vi "Main.vi"(11 "Module Admin":refnum<class "Delacor_lib_QMH_Module Admin.lvclass">) -> ()   [LabVIEW 2026, in "Launcher.lvlib"]
doc: "This template is based off of the Queued Message Handler design pattern and the Queued Message Handler project template that ships with LabVIEW.\n\nThe main difference is that the queue is private to this module and communication between modules is performed via Broadcast and Request events.\n\nRequest events are wrapped in public API methods and are handled in the Event Handling Loop (EHL) of this VI. Any module can register for Broadcast events sent by this module. The EHL generates messages based on user interface actions.\n\nThe Message Handling Loop (MHL) processes messages generated by the EHL, or by other messages. The messages are string values, so new messages can be added easily to the Message Cases case structure in the MHL. Each message cluster can also provide an optional value for Message Data, which is a variant that can be converted to whatever message-specific data is required.\n_____\nBased on DQMH Dev Tools: Project Template 7.1.2.1547."
uses:
  Launcher.lvlib
  <vilib>/Delacor/Delacor QMH/Libraries/Module Admin_class/Delacor_lib_QMH_Module Admin.lvclass
  Module Data--cluster.ctl
  Capture detection loop data--cluster.ctl
  <vilib>/Delacor/Delacor QMH/Libraries/Message Queue_class/Delacor_lib_QMH_Message Queue.lvclass/Delacor_lib_QMH_Message Queue.ctl
  Stop Argument--cluster.ctl
  <vilib>/Delacor/Delacor QMH/Libraries/Module Admin_class/Delacor_lib_QMH_Module Admin.lvclass/Delacor_lib_QMH_Module Admin.ctl
  Set Captures Folder Argument--cluster.ctl
  Set Capture Detection Loop Timeout Argument--cluster.ctl
  Trigger Capture Detection Loop Argument--cluster.ctl
  Trigger Capture Detection Loop (Reply Payload)--cluster.ctl
  <vilib>/Utility/miscctls.llb/LVPointTypeDef.ctl
  <vilib>/Delacor/Delacor QMH/Libraries/Message Queue_class/Delacor_lib_QMH_Enqueue Message (Single).vi
  <vilib>/Delacor/Delacor QMH/Libraries/Module Admin_class/Delacor_lib_QMH_Get External Launch.vi
  <vilib>/Delacor/Delacor QMH/Libraries/Message Queue_class/Delacor_lib_QMH_Message Queue.lvclass
  Core/Core.lvlib
panel:
  out "error out":errorcluster
  out "Status":string
  in  "Simulate MHL Error":bool
  in  "Simulate EHL Error":bool
  # "Other processes communicate with this Module via its Public API (wrappers for its Request Events).\n\nThis Module communicates with other processes via its Broadcast Events.\nAny process that wants to receive these messages can register for this module's Broadcast events."
  # "This template is for the DQMH framework. See the block diagram for more information on how to use this template."
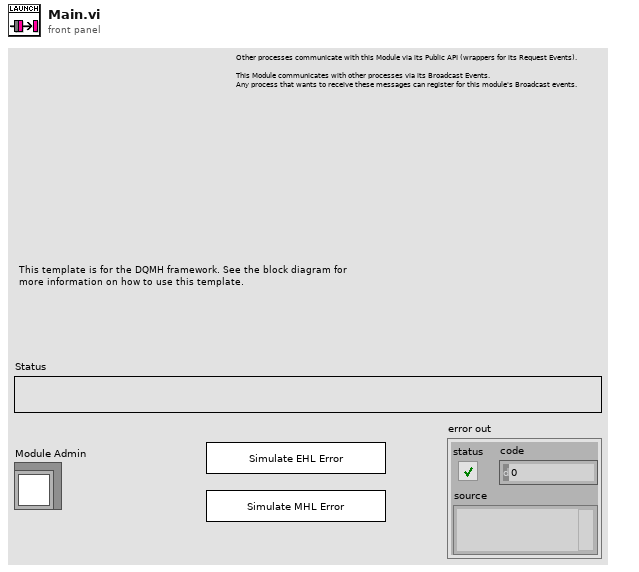
[diagram p1: front panel]
types:
  T1 = typedef "Launcher.lvlib/Broadcast Events--cluster.ctl" = cluster{"Module Did Init":refnum<user-event>, "Status Updated":refnum<user-event>, "Error Reported":refnum<user-event>, "Module Did Stop":refnum<user-event>, "Update Module Execution Status":refnum<user-event>, "Start Capture Detection Loop":refnum<user-event>, "Benchmark Started":refnum<user-event>, "Broadcast number of frames and run ID":refnum<user-event>}
  T2 = typedef "Launcher.lvlib/Request Events--cluster.ctl" = cluster{"Stop Module":refnum<user-event>, "Show Panel":refnum<user-event>, "Hide Panel":refnum<user-event>, "Get Module Execution Status":refnum<user-event>, "Show Diagram":refnum<user-event>, "Set Captures Folder":refnum<user-event>, "Set Capture Detection Loop Timeout":refnum<user-event>, "Trigger Capture Detection Loop":refnum<user-event>}
  T3 = typedef "Capture detection loop data--cluster.ctl" = cluster{"Captures":path, "Timeout":i32, "Reset":bool, "Trigger":bool, "Iteration":i32, "Capture":path}
  T4 = typedef "Launcher.lvlib/Module Data--cluster.ctl" = cluster{"Status":string, "Captures":path, "Capture Detection Loop Timeout":i32}
  T5 = enum32{"invalid lock state", "Not Locked", "Locked (No Password)", "Password-protected"}
  T6 = typedef "Launcher.lvlib/Stop Argument--cluster.ctl" = cluster{"Origin":string, "Exit via Stop Module Req?":bool, "Wait for Module to stop?":bool}
  T7 = typedef "Launcher.lvlib/Set Captures Folder Argument--cluster.ctl" = cluster{"Captures":path}
  T8 = typedef "Launcher.lvlib/Set Capture Detection Loop Timeout Argument--cluster.ctl" = cluster{"Timeout":i32}
  T9 = typedef "Launcher.lvlib/Trigger Capture Detection Loop Argument--cluster.ctl" = cluster{"Capture Detection Loop Timeout":i32, "Wait Notifier":refnum<notifier>, "wait for reply":bool}
  T10 = typedef "LVPointTypeDef.ctl" = cluster{"Horizontal":i16, "Vertical":i16}
  T11 = enum32{"Invalid", "Standard", "Closed", "Hidden", "Minimized", "Maximized"}
  T12 = typedef "Launcher.lvlib/Trigger Capture Detection Loop (Reply Payload)--cluster.ctl" = cluster{"Module Initial Time Stamp":timestamp, "error":errorcluster}
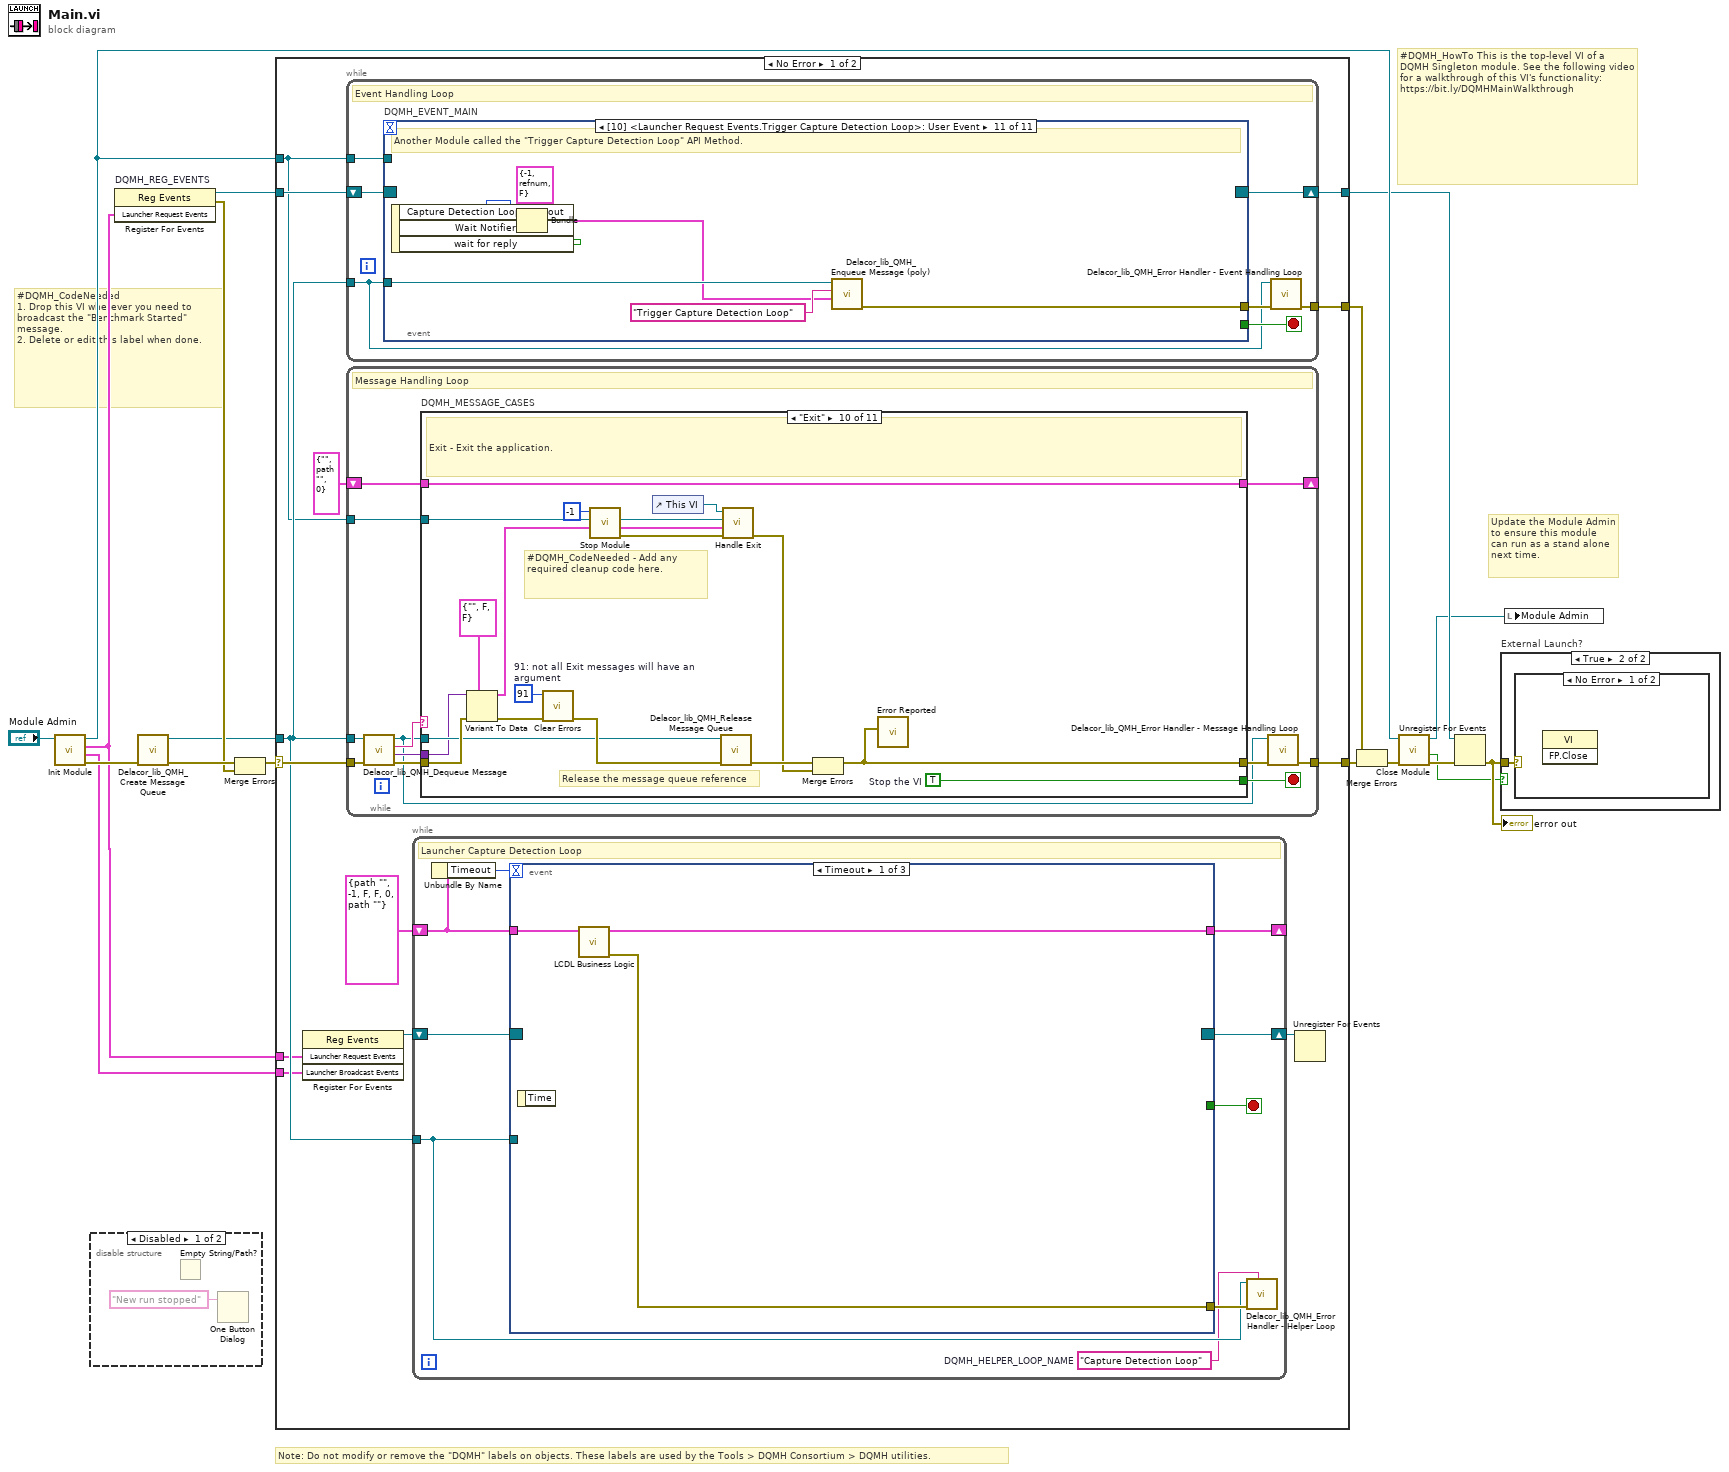
[diagram p0: block diagram]
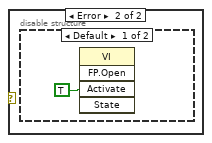
[diagram p4: hidden frame]
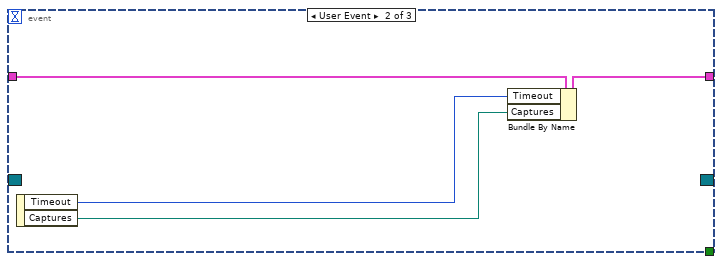
[diagram p6: hidden frame]
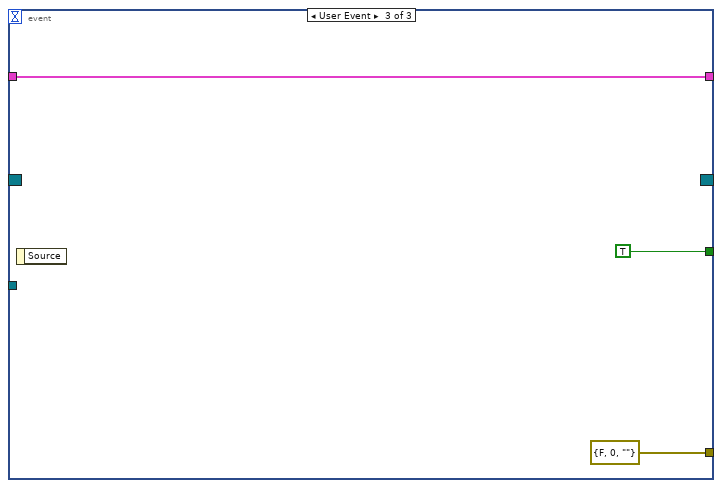
[diagram p7: hidden frame]
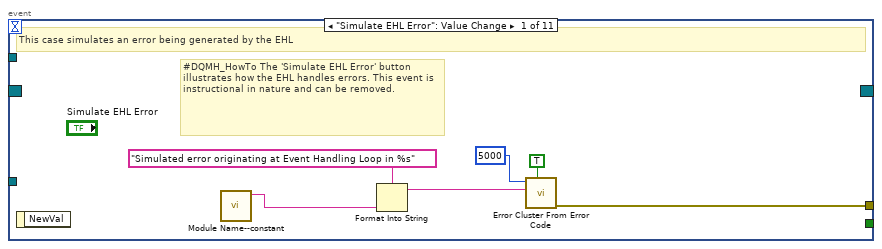
[diagram p8: hidden frame]
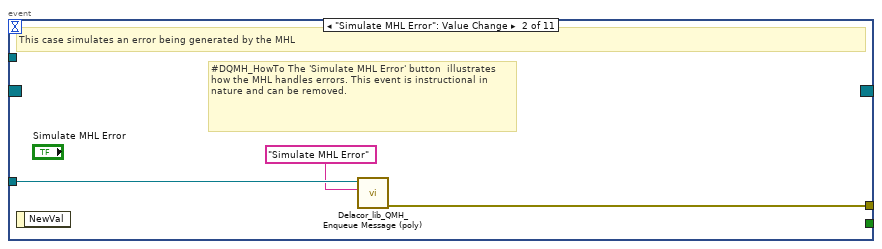
[diagram p9: hidden frame]
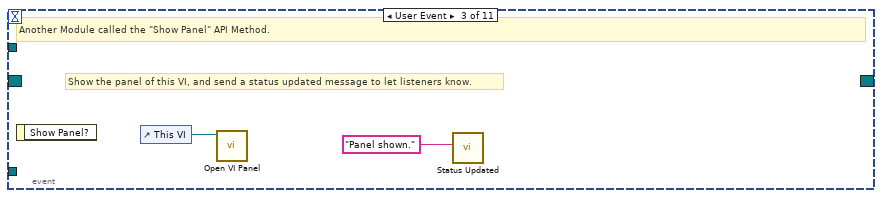
[diagram p10: hidden frame]
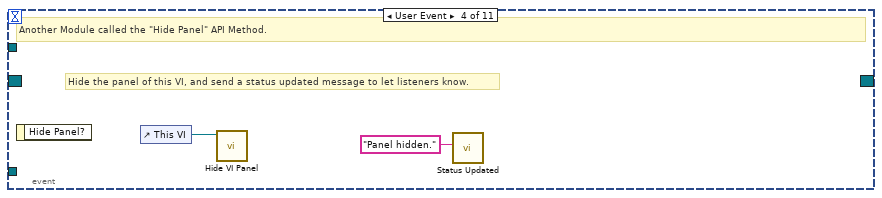
[diagram p11: hidden frame]
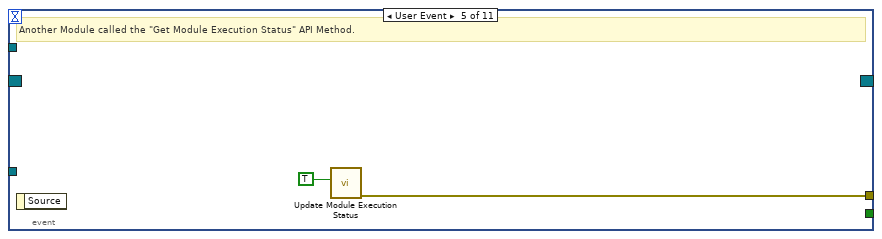
[diagram p12: hidden frame]
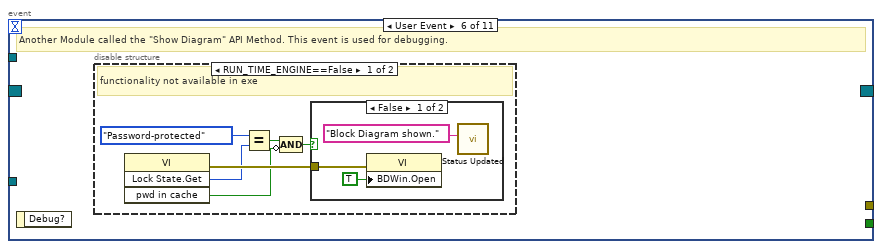
[diagram p13: hidden frame]
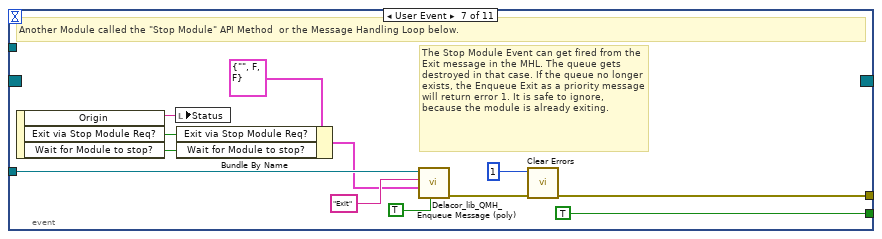
[diagram p16: hidden frame]
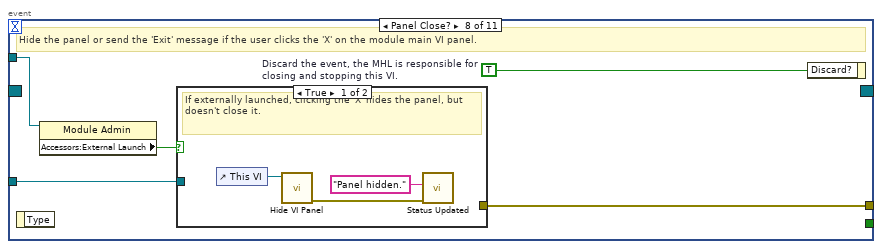
[diagram p17: hidden frame]
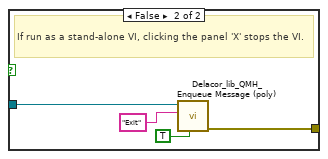
[diagram p18: hidden frame]
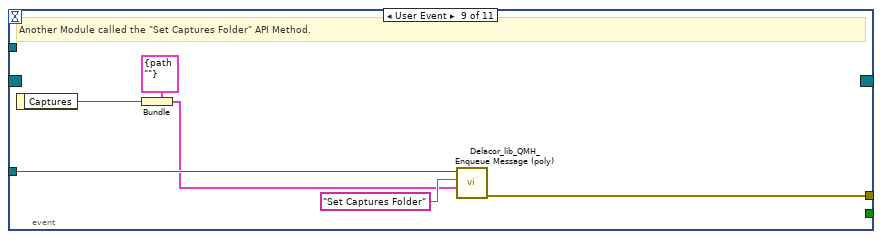
[diagram p19: hidden frame]
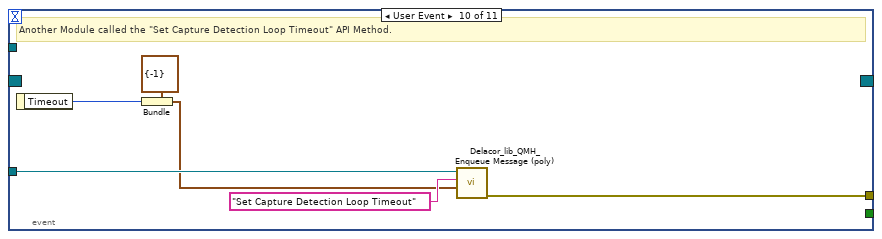
[diagram p20: hidden frame]
diagram:
  # "#DQMH_CodeNeeded\n1. Drop this VI wherever you need to broadcast the \"Broadcast Latest Frame\" message.\n2. Delete or edit this label when done."
  # "#DQMH_CodeNeeded\n1. Drop this VI wherever you need to broadcast the \"Benchmark Started\" message.\n2. Delete or edit this label when done."
  # "#DQMH_HowTo This is the top-level VI of a DQMH Singleton module. See the following video for a walkthrough of this VI's functionality: https://bit.ly/DQMHMainWalkthrough"
  # "Note: Do not modify or remove the \"DQMH\" labels on objects. These labels are used by the Tools > DQMH Consortium > DQMH utilities."
  # "Update the Module Admin to ensure this module can run as a stand alone next time."
  n1 = call "Init Module.vi"("Singleton Module Admin in"="Module Admin") -> ("error out"=w17:errorcluster, "Launcher Broadcast Events"=w1:T1, "Launcher Request Events"=w2:T2, "Singleton Module Admin out"=w9:refnum<class "Delacor_lib_QMH_Module Admin.lvclass">)  [unwired: 7 in]
  n2 = disable-structure shown="Disabled" {
    frame Disabled {
      n3 = Empty String/Path?() -> ()  [unwired: 1 in, 1 out]
      n4 = One Button Dialog(message="New run stopped") -> ()  [unwired: 1 in, 1 out]
    }
    frame Enabled {
    }
  }
  n5 = register-events "DQMH_REG_EVENTS"(w2) -> (reference out=w7:refnum<event-registration>, error out=w10:errorcluster)  [unwired: 2 in]
  n6 = call <vilib>:"Delacor_lib_QMH_Create Message Queue.vi"("error in"=w17) -> ("error out"=w12:errorcluster, "Message Queue"=w6:refnum<class "Delacor_lib_QMH_Message Queue.lvclass">)  [unwired: 9 in]
  n7 = Merge Errors(w12, w10) -> (w11:errorcluster)
  n8 = case shown="No Error" w11 {
    selector: w11 -> [w30 w259]
    tunnel: [w32 w258] -> w18
    tunnel: [w29 w257] -> w8
    tunnel: w7 -> [w27 w257]
    tunnel: w6 -> [w26 w252]
    tunnel: [w31 _] -> w15
    tunnel: w9 -> [w25 w253]
    tunnel: w2 -> [w24 _]
    tunnel: w1 -> [w21 _]
    frame No Error {
      n9 = register-events ("DQMH_HELPER_REGFOREVENTS")(w24, w21) -> (reference out=w22:refnum<event-registration>)  [unwired: 2 in, 1 out]
      n10 = while {
        tunnel: w26 -> [w52]
        shift-right: [w55] -> w29
        shift-left: w27 -> [w56]
        tunnel: [w57] -> w31
        tunnel: w25 -> [w53]
        stop <- w54 stop-if-true
        # "Event Handling Loop"
        n11 = event "DQMH_EVENT_MAIN" shown="[10] <Launcher Request Events.Trigger Capture Detection Loop>: User Event" {
          selector: w56 -> [_ _ _ _ _ _ _ _ _ _ _]
          dyn-events: [_ _ _ _ _ _ _ _ _ _ _] -> w55
          timeout: _ -> [_ _ _ _ _ _ _ _ _ _ _]
          tunnel: [_ _ _ _ _ _ TRUE ("Discard?") _ _ _ _] -> w54
          tunnel: w52 -> [_ w66 _ _ _ _ w90 w97 w112 w118 w126]
          tunnel: [w64 w67 _ _ w73 _ w93 w99 w107 w113 w119] -> w58
          tunnel: w53 -> [_ _ _ _ _ _ _ w96 _ _ _]
          event "Simulate EHL Error": Value Change {
            # "#DQMH_HowTo The 'Simulate EHL Error' button  illustrates how the EHL handles errors. This event is instructional in nature and can be removed."
            # "This case simulates an error being generated by the EHL"
            n12 = event-data() -> ()  [unwired: 1 in, 1 out]
            n13 = call "Module Name--constant.vi"() -> ("Module Name"=w61:string)  [unwired: 11 in]
            n14 = Format Into String(format string="Simulated error originating at Event Handling Loop in %s", w61) -> (resulting string=w62:string)  [unwired: 2 in, 1 out]
            n15 = call <vilib>:"Error Cluster From Error Code.vi"("show call chain? (False)"=TRUE, "error message (\"\")"=w62, "error code (0)"=5000) -> ("error out"=w64:errorcluster)  [unwired: 6 in]
          }
          event "Simulate MHL Error": Value Change {
            # "#DQMH_HowTo The 'Simulate MHL Error' button  illustrates how the MHL handles errors. This event is instructional in nature and can be removed."
            # "This case simulates an error being generated by the MHL"
            n16 = event-data() -> ()  [unwired: 1 in, 1 out]
            n17 = call-poly <vilib>:"Delacor_lib_QMH_Enqueue Message (poly).vi"("Message"="Simulate MHL Error", "Message Queue in"=w66) -> ("error out"=w67:errorcluster)  [unwired: 8 in, 1 out]
          }
          event User Event {
            # "Show the panel of this VI, and send a status updated message to let listeners know."
            # "Another Module called the \"Show Panel\" API Method."
            n18 = event-data() -> ()  [unwired: 1 in, 1 out]
            n19 = control-ref of="This VI"() -> (w69:refnum<vi>)
            n20 = call "Open VI Panel.vi"("VI"=w69) -> ()  [unwired: 10 in, 1 out]
            n21 = call "Status Updated.vi"("Status"="Panel shown." ("format string")) -> ()  [unwired: 10 in, 1 out]
          }
          event User Event {
            # "Hide the panel of this VI, and send a status updated message to let listeners know."
            # "Another Module called the \"Hide Panel\" API Method."
            n22 = event-data() -> ()  [unwired: 1 in, 1 out]
            n23 = control-ref of="This VI"() -> (w71:refnum<vi>)
            n24 = call "Hide VI Panel.vi"("VI"=w71) -> ()  [unwired: 10 in, 1 out]
            n25 = call "Status Updated.vi"("Status"="Panel hidden." ("format string")) -> ()  [unwired: 10 in, 1 out]
          }
          event User Event {
            # "Another Module called the \"Get Module Execution Status\" API Method."
            n26 = event-data() -> ()  [unwired: 1 in, 1 out]
            n27 = call "Update Module Execution Status.vi"("Running?"=TRUE) -> ("error out"=w73:errorcluster)  [unwired: 10 in]
          }
          event User Event {
            # "Another Module called the \"Show Diagram\" API Method. This event is used for debugging."
            n28 = event-data() -> ()  [unwired: 1 in, 1 out]
            n29 = disable-structure shown="RUN_TIME_ENGINE==False" {
              frame condition #0 (active) {
                # "functionality not available in exe"
                n30 = invoke on="Invoke Node" class="VI" method="Lock State.Get"() -> (error out=w79:errorcluster, "Get Lock State"=w78:T5, "pwd in cache"=w75:bool)  [unwired: 4 in, 1 out]
                n31 = Equal?(x=T5."Password-protected", y=w78) -> (x = y?=w76:bool)
                n32 = Compound Arithmetic op=AND(w76, invert w75) -> (w74:bool)
                n33 = case shown="False" w74 {
                  tunnel: w79 -> [w82 _]
                  frame False {
                    n34 = property on="Property Node" class="VI"(error in=w82, "BDWin.Open"=TRUE ("Block Diagram Window:Open")) -> ()  [unwired: 1 in, 2 out]
                    n35 = call "Status Updated.vi"("Status"="Block Diagram shown." ("format string")) -> ()  [unwired: 10 in, 1 out]
                  }
                  frame True {
                    # "Password-protected VI, and the password is not in the cache. Do not show the diagram."
                  }
                }
              }
              frame condition #1 {
              }
            }
          }
          event User Event {
            # "The Stop Module Event can get fired from the Exit message in the MHL. The queue gets destroyed in that case. If the queue no longer exists, the Enqueue Exit as a priority message will return error 1. It is safe to ignore, because the module is already exiting."
            # "Another Module called the \"Stop Module\" API Method  or the Message Handling Loop below."
            n36 = event-data() -> ("Origin"=w89:string, "Exit via Stop Module Req?"=w85:bool, "Wait for Module to stop?"=w84:bool)  [unwired: 1 in]
            n37 = local write "Status"(w89) -> ()
            n38 = Bundle By Name(cluster=T6 {"Origin"="", "Exit via Stop Module Req?"=FALSE, "Wait for Module to stop?"=FALSE} ("Stop Argument"), "Exit via Stop Module Req?"=w85, "Wait for Module to stop?"=w84) -> (w83:T6)
            n39 = call-poly <vilib>:"Delacor_lib_QMH_Enqueue Message (poly).vi"("Priority Message? (F)"=TRUE, "Message Data"=w83, "Message"="Exit", "Message Queue in"=w90) -> ("error out"=w94:errorcluster)  [unwired: 6 in, 1 out]
            n40 = call <vilib>:"Clear Errors.vi"("error in (no error)"=w94, "specific error code to clear (0: all)"=1) -> ("error out"=w93:errorcluster)  [unwired: 4 in, 1 out]
          }
          event Panel Close? {
            w98 = TRUE  # Discard the event, the MHL is responsible for closing and stopping this VI.
            # "Hide the panel or send the 'Exit' message if the user clicks the 'X' on the module main VI panel."
            n41 = event-data() -> ()  [unwired: 1 in, 1 out]
            n42 = property on="Property Node" class="Module Admin"(reference=w96) -> ("Accessors:External Launch"=w95:bool)  [unwired: 1 in, 2 out]
            n43 = case shown="True" w95 {
              tunnel: w97 -> [_ w105]
              tunnel: [_ w106] -> w99
              frame True {
                # "If externally launched, clicking the 'X' hides the panel, but doesn't close it."
                n44 = control-ref of="This VI"() -> (w102:refnum<vi>)
                n45 = call "Hide VI Panel.vi"("VI"=w102) -> ("error out"=w100:errorcluster)  [unwired: 10 in]
                n46 = call "Status Updated.vi"("error in"=w100, "Status"="Panel hidden." ("format string")) -> ()  [unwired: 9 in, 1 out]
              }
              frame False {
                # "If run as a stand-alone VI, clicking the panel 'X' stops the VI."
                n47 = call-poly <vilib>:"Delacor_lib_QMH_Enqueue Message (poly).vi"("Priority Message? (F)"=TRUE, "Message"="Exit", "Message Queue in"=w105) -> ("error out"=w106:errorcluster)  [unwired: 7 in, 1 out]
              }
            }
            n48 = event-data ("Event Filter Node")("Discard?"=w98) -> ()  [unwired: 1 in, 1 out]
          }
          event User Event {
            # "Another Module called the \"Set Captures Folder\" API Method."
            n49 = event-data() -> ("Captures"=w108:path)  [unwired: 1 in]
            n50 = Bundle(cluster=T7 {"Captures"=path ""} ("Set Captures Folder Argument"), "Captures"=w108) -> (w109:T7)
            n51 = call-poly <vilib>:"Delacor_lib_QMH_Enqueue Message (poly).vi"("Message Data"=w109, "Message"="Set Captures Folder", "Message Queue in"=w112) -> ("error out"=w107:errorcluster)  [unwired: 7 in, 1 out]
          }
          event User Event {
            # "Another Module called the \"Set Capture Detection Loop Timeout\" API Method."
            n52 = event-data() -> ("Timeout"=w114:i32)  [unwired: 1 in]
            n53 = Bundle(cluster=T8 {"Timeout"=-1} ("Set Capture Detection Loop Timeout Argument"), "Timeout"=w114) -> (w115:T8)
            n54 = call-poly <vilib>:"Delacor_lib_QMH_Enqueue Message (poly).vi"("Message Data"=w115, "Message"="Set Capture Detection Loop Timeout", "Message Queue in"=w118) -> ("error out"=w113:errorcluster)  [unwired: 7 in, 1 out]
          }
          event User Event {
            # "Another Module called the \"Trigger Capture Detection Loop\" API Method."
            n55 = event-data() -> ("Capture Detection Loop Timeout"=w122:i32, "Wait Notifier"=w121:refnum<notifier>, "wait for reply"=w120:bool)  [unwired: 1 in]
            n56 = Bundle(cluster=T9 {"Capture Detection Loop Timeout"=-1, "Wait Notifier"=refnum, "wait for reply"=FALSE} ("Trigger Capture Detection Loop Argument"), "Capture Detection Loop Timeout"=w122, "Wait Notifier"=w121, "wait for reply"=w120) -> (w123:T9)
            n57 = call-poly <vilib>:"Delacor_lib_QMH_Enqueue Message (poly).vi"("Message Data"=w123, "Message"="Trigger Capture Detection Loop", "Message Queue in"=w126) -> ("error out"=w119:errorcluster)  [unwired: 7 in, 1 out]
          }
        }
        n58 = call-dynamic "Delacor_lib_QMH_Error Handler - Event Handling Loop.vi"("error in"=w58, "Message Queue in"=w52) -> ("dup error in"=w57:errorcluster)  [unwired: 8 in, 1 out]
      }
      n59 = while {
        tunnel: w26 -> [w127]
        shift-right: [w135] -> _
        shift-left: T4 {"Status"="", "Captures"=path "", "Capture Detection Loop Timeout"=0} ("Data Cluster") -> [w136]
        tunnel: w30 -> [w138]
        tunnel: [w130] -> w32
        tunnel: w25 -> [w131]
        stop <- w134 stop-if-true
        # "Message Handling Loop"
        n60 = call-dynamic "Delacor_lib_QMH_Dequeue Message.vi"("error in"=w138, "Message Queue in"=w127) -> ("error out"=w137:errorcluster, "Message Data"=w132:variant, "Message"=w133:string, "Message Queue out"=w128:refnum<class "Delacor_lib_QMH_Message Queue.lvclass">)  [unwired: 6 in]
        n61 = case "DQMH_MESSAGE_CASES" shown="\"Exit\"" w133 {
          selector: w133 -> [_ _ _ _ _ _ _ _ _ _ w247]
          tunnel: w128 -> [_ _ _ _ _ _ _ _ w211 w235 _]
          tunnel: w137 -> [w156 w160 w170 w179 w191 w196 w198 w207 w218 w241 w250]
          tunnel: [w154 w160 w164 w174 w182 w195 w198 w206 w214 w236 w251] -> w129
          tunnel: w136 -> [w145 w159 w162 w172 w190 w194 w197 w204 w213 w234 w248]
          tunnel: [w144 w159 w166 w172 w190 w194 w197 w204 w213 w234 w248] -> w135
          tunnel: [_ _ _ _ _ _ _ _ _ w233 _] -> w134
          tunnel: w132 -> [_ _ w169 w178 w189 _ _ _ w212 w232 _]
          tunnel: w131 -> [w146 _ _ _ _ _ _ _ w210 w227 _]
          frame "Initialize" {
            w140 = "Initial Message" ("Initial Message")
            # "#DQMH_CodeNeeded - Initialize the appearance of the front panel."
            # "#DQMH_CodeNeeded - Initialize your state data here."
            # "Initialize - Any operation that needs to be done before the module can receive messages. Synchronize Caller Events.vi will inform Start Module.vi that the module has launched and is ready to receive messages. Module Did Init.vi will broadcast that the module initialized."
            n62 = call "Synchronize Caller Events.vi"("error in"=w156, "Singleton Module Admin in"=w146) -> ("error out"=w155:errorcluster, "Singleton Module Admin out"=w141:refnum<class "Delacor_lib_QMH_Module Admin.lvclass">)  [unwired: 8 in]
            n63 = property on="Property Node" class="Module Admin"(reference=w141) -> ("Accessors:External Launch"=w150:bool)  [unwired: 1 in, 2 out]
            n64 = Select(t=T11."Hidden" ("State"), s=w150, f=T11."Standard" ("State")) -> (s? t:f=w147:T11)
            n65 = call "Module Name--constant.vi"() -> ("Module Name"=w153:string)  [unwired: 11 in]
            n66 = property on="Property Node" class="VI"("Front Panel.Title"=w153) -> (reference out=w152:refnum<vi>, error out=w158:errorcluster)  [unwired: 2 in]
            n67 = invoke on="Invoke Node" class="VI" method="FP.Open"(reference=w152, error in=w158, "State"=w147) -> (reference out=w151:refnum<vi>, error out=w157:errorcluster)  [unwired: 2 in, 3 out]
            n68 = Bundle By Name(cluster=w145, "Status"=w140) -> (w144:T4)
            n69 = invoke on="Invoke Node" class="VI" method="FP.Center"(reference=w151, error in=w157) -> ()  [unwired: 1 in, 3 out]
            n70 = property on="Pane" class="Pane"("Origin"=T10 {"Horizontal"=0, "Vertical"=0}) -> ()  [unwired: 2 in, 2 out]
            n71 = call "Module Name--constant.vi"() -> ("Module Name"=w142:string)  [unwired: 11 in]
            n72 = call "Module Did Init.vi"("error in"=w155, "Initialized?"=TRUE, "Origin"=w142) -> ("error out"=w154:errorcluster)  [unwired: 8 in]
            "Status" <- w140
          }
          frame "---Module Specific---" {
            # "Separator -- The following cases handle messages specific to this Module."
          }
          frame "Set Captures Folder" {
            n73 = Variant To Data(error in=w170, type=T7 {"Captures"=path ""} ("Set Captures Folder Argument"), Variant=w169) -> (data=w167:T7, error out=w165:errorcluster)
            n74 = Unbundle By Name(w167) -> ("Captures"=w161:path)
            n75 = Unbundle By Name(w162) -> ("Capture Detection Loop Timeout"=w163:i32)
            n76 = Bundle By Name(cluster=w162, "Captures"=w161) -> (w166:T4)
            n77 = call "Start Capture Detection Loop.vi"("error in"=w165, "Captures"=w161, "Timeout"=w163) -> ("error out"=w164:errorcluster)  [unwired: 8 in]
          }
          frame "Set Capture Detection Loop Timeout" {
            # "#DQMH_CodeNeeded\n1. Configure this Message Case for handling the \"Set Capture Detection Loop Timeout\" message.\n2. Delete or edit this label when done."
            n78 = Variant To Data(error in=w179, type=T8 {"Timeout"=-1} ("Set Capture Detection Loop Timeout Argument"), Variant=w178) -> (data=w176:T8, error out=w175:errorcluster)
            n79 = Unbundle By Name(w176) -> ("Timeout"=w173:i32)
            n80 = Unbundle By Name(w172) -> ("Captures"=w171:path)
            n81 = call "Start Capture Detection Loop.vi"("error in"=w175, "Captures"=w171, "Timeout"=w173) -> ("error out"=w174:errorcluster)  [unwired: 8 in]
          }
          frame "Trigger Capture Detection Loop" {
            (unwired) 0  # Capture Detection Loop Timeout
            # "#DQMH_CodeNeeded\n1. Configure this Message Case for handling the \"Trigger Capture Detection Loop\" message.\n2. Wire any error that occurs to the \"error\" terminal.\n3. Delete or edit this label when done."
            n82 = Variant To Data(error in=w191, type=T9 {"Capture Detection Loop Timeout"=-1, "Wait Notifier"=refnum, "wait for reply"=FALSE} ("Trigger Capture Detection Loop Argument"), Variant=w189) -> (data=w187:T9, error out=w180:errorcluster)
            n83 = Unbundle By Name(w187) -> ("Wait Notifier"=w186:refnum<notifier>, "wait for reply"=w185:bool)  [unwired: 1 out]
            n84 = Get Date/Time In Seconds() -> (seconds since 1Jan1904=w181:timestamp)
            n85 = Bundle By Name(cluster=T12 {"Module Initial Time Stamp"=timestamp(0 s since 1904-01-01), "error"={"status"=FALSE, "code"=0, "source"=""}} ("Trigger Capture Detection Loop (Reply Payload)"), "Module Initial Time Stamp"=w181, "error"=w180) -> (w184:T12)
            n86 = Merge Errors(w180) -> (w182:errorcluster)
            n87 = case "DQMH_FIRE_NOTIFIER" shown="True" w185 {
              tunnel: w186 -> [_ w193]
              tunnel: w184 -> [_ w192]
              frame False {
              }
              frame True {
                n88 = Send Notification(notification=w192, notifier=w193) -> ()  [unwired: 1 in, 2 out]
              }
            }
          }
          frame "---Copy This Frame---" {
            # "Duplicate this frame when creating new messages.  Change this comment in the duplicated frame to describe this message."
            n89 = Merge Errors(w196) -> (w195:errorcluster)
          }
          frame "---Exit and Error Handling---" {
            # "Separator - The following cases handle errors and exit messages."
          }
          frame "Simulate MHL Error" {
            # "#DQMH_HowTo The 'Simulate MHL Error' button  illustrates how the MHL handles errors. This event is instructional in nature and can be removed."
            # "Simulate an error occurring at the MHL"
            n90 = call "Module Name--constant.vi"() -> ("Module Name"=w200:string)  [unwired: 11 in]
            n91 = Format Into String(format string="Simulated error originating at Message Handling Loop in %s", w200) -> (resulting string=w201:string)  [unwired: 2 in, 1 out]
            n92 = call <vilib>:"Error Cluster From Error Code.vi"("show call chain? (False)"=TRUE, "error message (\"\")"=w201, "error code (0)"=5001) -> ("error out"=w205:errorcluster)  [unwired: 6 in]
            n93 = Merge Errors(w207, w205) -> (w206:errorcluster)
          }
          frame "Error" {
            # "#DQMH_CodeRecommended - If the module is running in standalone mode (External Launch = FALSE), this code will pop up an error dialog and call the 'Exit' message if an error occurs. Add more fine-grained error management here."
            # "Error - Check the error message data and respond accordingly. This message is sent by the \"Error Handler\" VIs at the end of each loop in this application."
            n94 = property on="Property Node" class="Module Admin"(reference=w210) -> ("Accessors:External Launch"=w209:bool)  [unwired: 1 in, 2 out]
            n95 = Variant To Data(error in=w218, type=errorcluster {"status"=FALSE, "code"=0, "source"=""} ("error constant"), Variant=w212) -> (data=w208:errorcluster, error out=w216:errorcluster)
            n96 = local write "error out"(w208) -> ()
            n97 = call "Error Reported.vi"("Error"=w208) -> ()  [unwired: 10 in, 1 out]
            n98 = case shown="False" w209 {
              tunnel: [w223 _] -> w215
              tunnel: w211 -> [w221 _]
              tunnel: w208 -> [w222 _]
              frame False {
                n99 = disable-structure shown="Default" {
                  disable-tunnel: w222 -> [w224 _]
                  frame condition #0 (active) {
                    # "If the module is running standalone, then pop up an error dialog and call the \"Exit\" message."
                    n100 = call <vilib>:"Simple Error Handler.vi"("error in (no error)"=w224) -> ()  [unwired: 4 in, 5 out]
                  }
                  frame condition #1 {
                    # "To prevent the Simple Error Handler VI from being loaded (e.g. when deploying to a Real-Time target), add the Conditional Disable Symbol \"DQMH_Disable_SEH\" to your project and set it to TRUE."
                  }
                }
                n101 = call-poly <vilib>:"Delacor_lib_QMH_Enqueue Message (poly).vi"("Priority Message? (F)"=TRUE, "Message"="Exit", "Message Queue in"=w221) -> ("error out"=w223:errorcluster)  [unwired: 7 in, 1 out]
              }
              frame True {
                # "If the module was launched externally, calling the Error Reported broadcast VI is the only action performed by the \"Error\" message. The module's caller can then process the error appropriately."
              }
            }
            n102 = Merge Errors(w216, w215) -> (w214:errorcluster)
          }
          frame "Exit" {
            w231 = 91  # 91: not all Exit messages will have an argument
            w233 = TRUE  # Stop the VI
            # "Release the message queue reference"
            # "#DQMH_CodeNeeded - Add any required cleanup code here."
            # "Exit - Exit the application."
            n103 = Variant To Data(error in=w241, type=T6 {"Origin"="", "Exit via Stop Module Req?"=FALSE, "Wait for Module to stop?"=FALSE} ("Stop Argument"), Variant=w232) -> (data=w229:T6, error out=w238:errorcluster)
            n104 = call <vilib>:"Clear Errors.vi"("error in (no error)"=w238, "specific error code to clear (0: all)"=w231) -> ("error out"=w240:errorcluster)  [unwired: 4 in, 1 out]
            n105 = call "Stop Module.vi"("Module ID"=-1) -> ("error out"=w226:errorcluster)  [unwired: 10 in]
            n106 = control-ref of="This VI"() -> (w228:refnum<vi>)
            n107 = call-dynamic "Delacor_lib_QMH_Release Message Queue.vi"("error in"=w240, "Message Queue"=w235) -> ("error out"=w239:errorcluster)  [unwired: 9 in]
            n108 = call "Handle Exit.vi"("error in"=w226, "Stop Argument"=w229, "Admin in"=w227, "VI reference"=w228) -> ("error out"=w237:errorcluster)  [unwired: 6 in, 1 out]
            n109 = Merge Errors(w239, w237) -> (w236:errorcluster)
            n110 = call "Error Reported.vi"("Error"=w236) -> ()  [unwired: 10 in, 1 out]
          }
          frame Default {
            # "'Default' case only runs if there is a message that isn't defined in any of the other cases.  Output a programming error."
            n111 = call "Module Name--constant.vi"() -> ("Module Name"=w246:string)  [unwired: 11 in]
            n112 = Format Into String(format string="The invalid message string \"%s\" was received in the Message Handling Loop for module \"%s\".", w247, w246) -> (resulting string=w242:string)  [unwired: 2 in, 1 out]
            n113 = call <vilib>:"Error Cluster From Error Code.vi"("show call chain? (False)"=TRUE, "error message (\"\")"=w242, "error code (0)"=1) -> ("error out"=w249:errorcluster)  [unwired: 6 in]
            n114 = Merge Errors(w250, w249) -> (w251:errorcluster)
          }
        }
        n115 = call-dynamic "Delacor_lib_QMH_Error Handler - Message Handling Loop.vi"("error in"=w129, "Message Queue in"=w128) -> ("dup error in"=w130:errorcluster)  [unwired: 8 in, 1 out]
      }
      n116 = while "DQMH_HELPER_LOOP" {
        shift-right: [w40] -> w23
        shift-left: w22 -> [w41]
        tunnel: w26 -> [w37]
        shift-right: [w33] -> _
        shift-left: T3 {"Captures"=path "", "Timeout"=-1, "Reset"=FALSE, "Trigger"=FALSE, "Iteration"=0, "Capture"=path ""} ("CaptureDetectionLoopData") -> [w34]
        stop <- w39 stop-if-true
        w36 = "Capture Detection Loop"  # DQMH_HELPER_LOOP_NAME
        # "Launcher Capture Detection Loop"
        n117 = Unbundle By Name(w34) -> ("Timeout"=w35:i32)
        n118 = event "DQMH_HELPER_EVENT_STRUCTURE" shown="[0] Timeout" {
          selector: w41 -> [_ _ _]
          dyn-events: [_ _ _] -> w40
          timeout: w35 -> [_ _ _]
          tunnel: [_ _ TRUE] -> w39
          tunnel: [w42 _ errorcluster {"status"=FALSE, "code"=0, "source"=""} ("error constant")] -> w38
          tunnel: w37 -> [_ _ _]
          tunnel: w34 -> [w44 w48 w49]
          tunnel: [w43 w46 w49] -> w33
          event Timeout {
            n119 = event-data() -> ()  [unwired: 1 in, 1 out]
            n120 = call "LCDL Business Logic.vi"("CaptureDetectionLoopDataIn"=w44) -> ("error out"=w42:errorcluster, "CaptureDetectionLoopDataOut"=w43:T3)  [unwired: 8 in, 1 out]
          }
          event User Event {
            n121 = event-data() -> ("Timeout"=w45:i32, "Captures"=w47:path)  [unwired: 1 in]
            n122 = Bundle By Name(cluster=w48, "Timeout"=w45, "Captures"=w47) -> (w46:T3)
          }
          event User Event {
            n123 = event-data() -> ()  [unwired: 1 in, 1 out]
          }
        }
        n124 = call-dynamic "Delacor_lib_QMH_Error Handler - Helper Loop.vi"("Error Debug"=w36, "error in"=w38, "Message Queue in"=w37) -> ()  [unwired: 7 in, 2 out]
      }
      n125 = Unregister For Events(event registration refnum=w23) -> ()  [unwired: 1 in, 1 out]
    }
    frame Error {
      # "Synchronize Caller Events.vi will inform Start Module.vi that the module has launched and will let the code calling Start Module.vi register for broadcasts and would permit the caller receive the broadcast that an error occurred at launch time."
      n126 = call-dynamic "Delacor_lib_QMH_Release Message Queue.vi"("error in"=w259, "Message Queue"=w252) -> ("error out"=w258:errorcluster)  [unwired: 9 in]
      n127 = call "Synchronize Caller Events.vi"("Singleton Module Admin in"=w253) -> ("error out"=w260:errorcluster)  [unwired: 9 in, 1 out]
      n128 = call "Module Name--constant.vi"() -> ("Module Name"=w256:string)  [unwired: 11 in]
      n129 = Format Into String(format string="An error occurred during initialization. %s is no longer running.", w256) -> (resulting string=w254:string)  [unwired: 2 in, 1 out]
      n130 = Merge Errors(w258, w260) -> (w261:errorcluster)
      n131 = call "Error Reported.vi"("Additional Information"=w254, "Error"=w261) -> ()  [unwired: 9 in, 1 out]
    }
  }
  n132 = Merge Errors(w15, w18) -> (w14:errorcluster)
  n133 = call "Close Module.vi"("error in"=w14, "Module Admin in"=w9) -> ("error out"=w16:errorcluster, "External Launch"=w3:bool, "Module Admin out"=w4:refnum<class "Delacor_lib_QMH_Module Admin.lvclass">)  [unwired: 7 in]
  n134 = Unregister For Events(event registration refnum=w8, error in=w16) -> (error out=w13:errorcluster)
  "error out" <- w13
  n135 = case "External Launch?" shown="True" w3 {
    tunnel: w13 -> [_ w262]
    frame False {
    }
    frame True {
      n136 = case shown="No Error" w262 {
        frame No Error {
          n137 = invoke on="Invoke Node" class="VI" method="FP.Close"() -> ()  [unwired: 3 in, 3 out]
        }
        frame Error {
          n138 = disable-structure shown="Default" {
            frame condition #0 (active) {
              n139 = invoke class="VI" method="FP.Open"("Activate"=TRUE ("Activate?")) -> ()  [unwired: 4 in, 5 out]
            }
            frame condition #1 {
              # "Don't show panel on error if running inside a built EXE."
            }
          }
        }
      }
    }
  }
  n140 = local write "Module Admin"(w4) -> ()
